vi "Get as LabVIEW Text.vi"(8 "error in (no error)":errorcluster, 10 "Name Array":string[](array[string]), 11 "JSON Scalar in":refnum<class "JSON Scalar.lvclass">) -> (0 "error out":errorcluster, 2 "LabVIEW Text":string, 3 "JSON Scalar out":refnum<class "JSON Scalar.lvclass">)   [LabVIEW 2011, in "JSON Scalar.lvclass"]
uses:
  JSON Scalar.lvclass
  JSON Scalar.lvclass/JSON Scalar.ctl
  JSON Value/JSON Value.lvclass
panel:
  # "Value formated as LabVIEW text:\n-- no quotes on JSON strings\n-- LabVIEW text encoding <ToDo>\n-- no escaped characters <ToDo>"
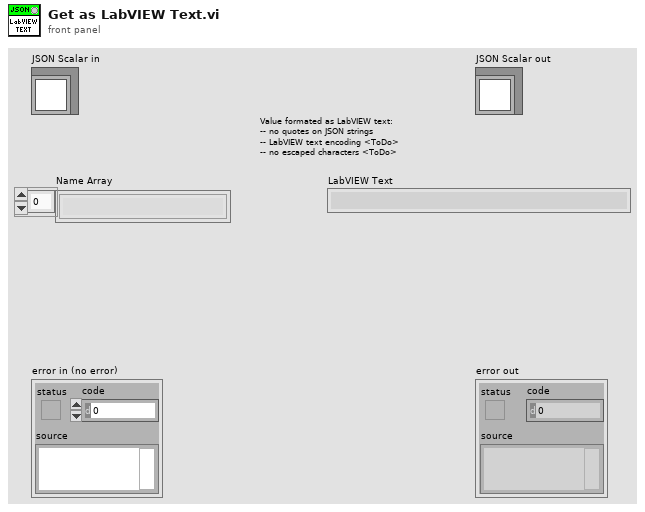
[diagram p1: front panel]
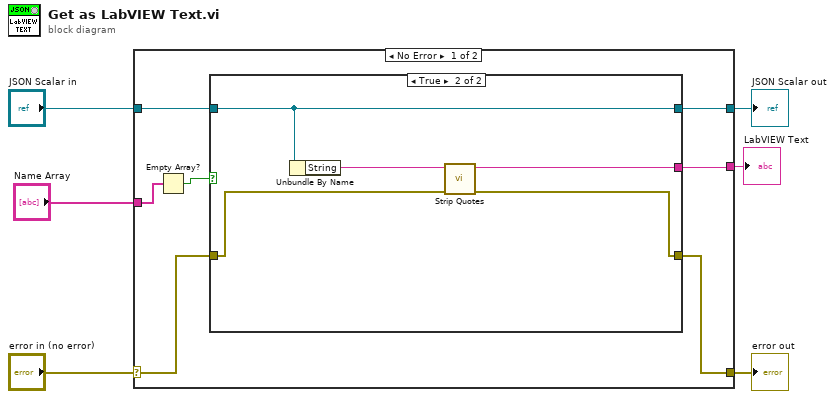
[diagram p0: block diagram]
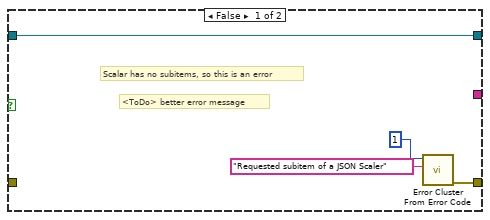
[diagram p2: hidden frame]
diagram:
  n1 = case shown="No Error" "error in (no error)" {
    selector: "error in (no error)" -> [w8 w24]
    tunnel: [w7 w24] -> w5
    tunnel: [w9 w23] -> w3
    tunnel: "JSON Scalar in" -> [w10 w23]
    tunnel: [w13 _] -> w2
    tunnel: "Name Array" -> [w12 _]
    frame No Error {
      n2 = Empty Array?(array=w12) -> (empty?=w11:bool)
      n3 = case shown="True" w11 {
        tunnel: w10 -> [w17 w20]
        tunnel: [_ w21] -> w13
        tunnel: [w17 w20] -> w9
        tunnel: w8 -> [_ w19]
        tunnel: [w16 w18] -> w7
        frame False {
          # "<ToDo> better error message"
          # "Scalar has no subitems, so this is an error"
          n4 = call <vilib>:"Error Cluster From Error Code.vi"("error message (\"\")"="Requested subitem of a JSON Scaler" ("error message (\"\")"), "error code (0)"=1) -> ("error out"=w16:errorcluster)  [unwired: 7 in]
        }
        frame True {
          n5 = Unbundle By Name(w20) -> ("String"=w22:string)
          n6 = call "Strip Quotes.vi"("error in (no error)"=w19, "String"=w22) -> ("error out"=w18:errorcluster, "result string"=w21:string)  [unwired: 8 in]
        }
      }
    }
    frame Error {
    }
  }
  "error out" <- w5
  "JSON Scalar out" <- w3
  "LabVIEW Text" <- w2
